vi "Knock Cylinder 1.0 FPGA Inputs Write Node.vi"(8 "error in (no error)":errorcluster, 10 "input":T2, 11 "Refnum in":T1) -> (0 "error out":errorcluster, 3 "Refnum out":T1)   [LabVIEW 2019, in "Engine Simulation Toolkit Engine.lvlib"]
uses:
  Engine Simulation Toolkit Engine.lvlib
  Knock Cylinder 1.0 Input Ref.ctl
  <vilib>/Utility/error.llb/Error Cluster From Error Code.vi
  <vilib>/rvi/errors/niLvFpgaAdjustHostInterfaceError.vi
  <vilib>/rvi/interface/nirviReadWriteControl/nirviReadWriteControl.xnode
  NiFpgaLv.dll
  <vilib>/rvi/interface/Simulation/niFpgaSimulationCallBeginRW.vi
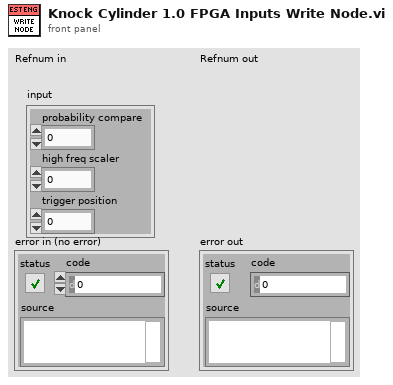
[diagram p1: front panel]
types:
  T1 = typedef "Engine Simulation Toolkit Engine.lvlib/Knock Cylinder 1.0 Input Ref.ctl" = refnum<k20>
  T2 = cluster{"probability compare":u16, "high freq scaler":fxp<+,10,0>, "trigger position":u16}
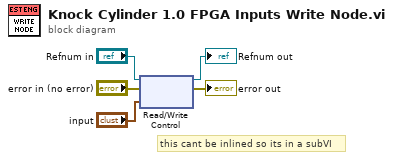
[diagram p0: block diagram]
diagram:
  # "this cant be inlined so its in a subVI"
  n1 = xnode "Read/Write Control"("FPGA VI Reference In"="Refnum in", "error in"="error in (no error)", "Value"="input") -> ("FPGA VI Reference Out"=→"Refnum out":T1, "error out"=→"error out":errorcluster)
